vi "LVIS_VerifyConfig.vi"(8 "Error In":errorcluster) -> (0 "Error Out":errorcluster)   [LabVIEW 2015]
doc: "Verifies the LVIS_Settings file configuration values for the Event, Test and Measurement parameters."
uses:
  Globals/LVIS_IsGlobal.vi
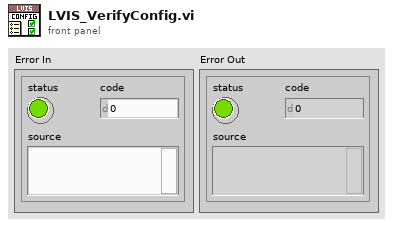
[diagram p1: front panel]
types:
  T1 = cluster{"EventName":string, "EventStart":string, "EventStop":string, "EventStatus":string, "EventClientID":string, "IS_EventID":string, "EventMeta":string, "ProductLine":string, "ProcessName":string, "Station":string, "Operator":string, "SN":string, "Model":string, "Manufacturer":string}
  T2 = cluster{"[0]":string, "[1]":string, "[2]":string, "[3]":string, "[4]":string, "[5]":string, "[6]":string, "[7]":string, "[8]":string, "[9]":string, "[10]":string, "[11]":string, "[12]":string, "[13]":string}
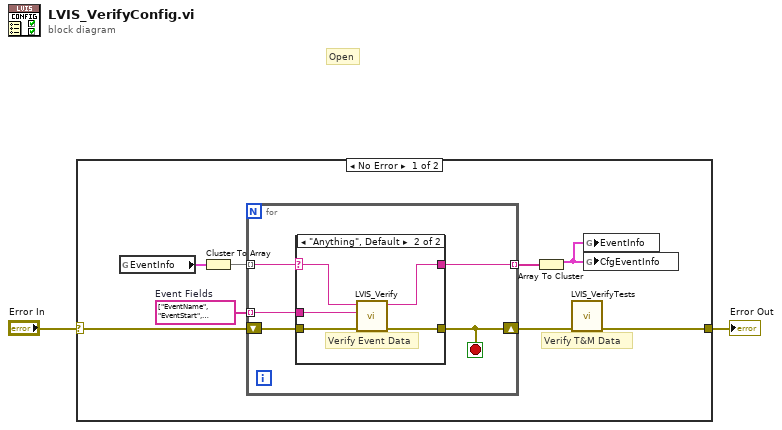
[diagram p0: block diagram]
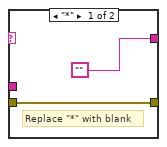
[diagram p2: hidden frame]
diagram:
  # "Open"
  n1 = case shown="No Error" "Error In" {
    selector: "Error In" -> [w10 w23]
    tunnel: [w4 w23] -> w1
    frame No Error {
      w7 = string[] ["EventName", "EventStart", "EventStop", "EventStatus", "EventClientID", "IS_EventID", "EventMeta", "ProductLine", "ProcessName", "Station", "Operator", "SN", "Model", "Manufacturer"]  # Event Fields
      # "Verify T&M Data"
      n2 = global read "LVIS_IsGlobal.vi" "EventInfo"() -> (w9:T1)
      n3 = Cluster To Array(cluster=w9) -> (array=w8:string[])
      n4 = for {
        tunnel: w8 -> [w13] mode=indexing
        tunnel: w7 -> [w14] mode=indexing
        shift-right: [w11] -> w5
        shift-left: w10 -> [w15]
        tunnel: [w12] -> w6 mode=indexing
        stop <- w11 stop-if-true
        n5 = case shown="\"Anything\", Default" w13 {
          selector: w13 -> [_ w19]
          tunnel: w15 -> [w17 w22]
          tunnel: [w17 w21] -> w11
          tunnel: ["" w18] -> w12
          tunnel: w14 -> [_ w20]
          frame "*" {
            # "Replace \"*\" with blank"
          }
          frame "Anything", Default {
            # "Verify Event Data"
            n6 = call "LVIS_Verify.vi"("Error In"=w22, "Field Name"=w20, "Field Value In"=w19) -> ("Error Out"=w21:errorcluster, "Field Value Out"=w18:string)  [unwired: 7 in]
          }
        }
      }
      n7 = Array To Cluster(array=w6) -> (cluster=w3:T2)
      n8 = call "LVIS_VerifyTests.vi"("Error In"=w5) -> ("Error Out"=w4:errorcluster)  [unwired: 10 in]
      n9 = global write "LVIS_IsGlobal.vi" "EventInfo"(w3) -> ()
      n10 = global write "LVIS_IsGlobal.vi" "CfgEventInfo"(w3) -> ()
    }
    frame Error {
    }
  }
  "Error Out" <- w1
